vi "capt_scaling.vi"(8 "error in":errorcluster, 10 "Gain":sgl format="%.6e", 11 "Offset":sgl format="%.6e") -> (0 "error out":errorcluster)   [LabVIEW 2012]
panel:
  in  "Address":u8=250 format="%x"
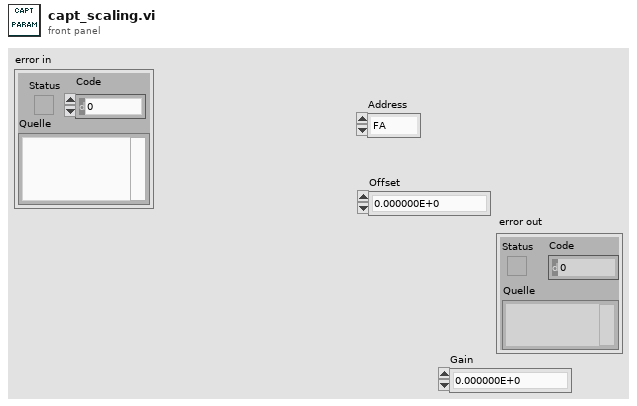
[diagram p1: front panel]
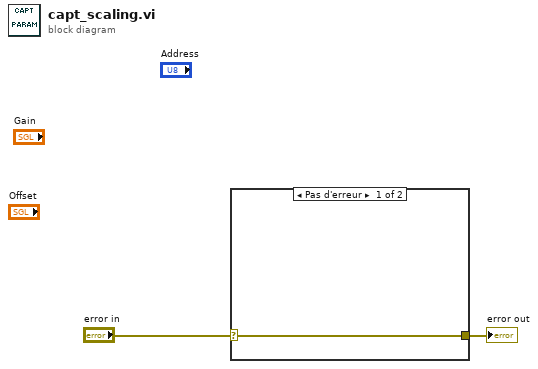
[diagram p0: block diagram]
diagram:
  n1 = case shown="Pas d'erreur" "error in" {
    selector: "error in" -> [w3 w4]
    tunnel: [w3 w4] -> w2
    frame No Error {
    }
    frame Error {
    }
  }
  "error out" <- w2
